vi "Map Tags to Channels.vi"(7 "instance id":string, 8 "error in (no error)":errorcluster, 9 "String Array":string[][](array[string]), 10 "Lines":T1[](array[typedef]), 11 "engine configuration in":refnum<class "engine configuration.lvclass">) -> (0 "error out":errorcluster, 3 "engine configuration out":refnum<class "engine configuration.lvclass">)   [LabVIEW 2018, in "Benchmark PID editor node.lvclass"]
uses:
  Benchmark PID editor node.lvclass
  module/configuration/Line.ctl
  <vilib>/NI/Tag Bus Module Framework/channel/TBM channel.lvclass
  C:/Program Files (x86)/National Instruments/LabVIEW 2018/vi.lib/NI/Tag Bus/tag/tag descriptor.lvclass
  <vilib>/NI/Module Execution Interface/Engine Configuration/engine configuration.lvclass
  <vilib>/NI/Tag Bus/tag/tag descriptor.lvclass/tag descriptor.ctl
  <vilib>/NI/Tag Bus/tag/tag descriptor.lvclass
  module/configuration/Benchmark PID configuration.lvclass
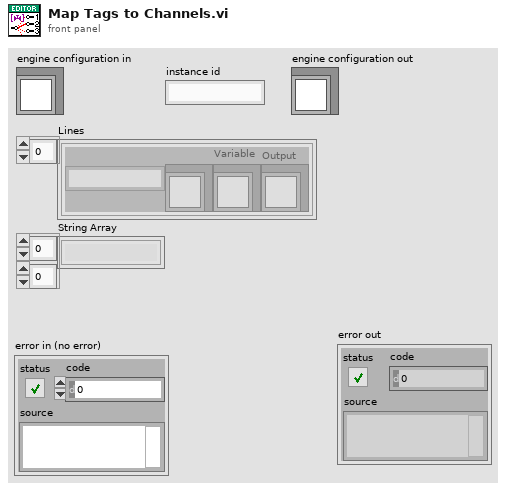
[diagram p1: front panel]
types:
  T1 = typedef "Benchmark PID configuration.lvclass/Line.ctl" = cluster{"PID Name":string, "Setpoint":refnum<class "TBM channel.lvclass">, "Variable":refnum<class "TBM channel.lvclass">, "Output":refnum<class "TBM channel.lvclass">}
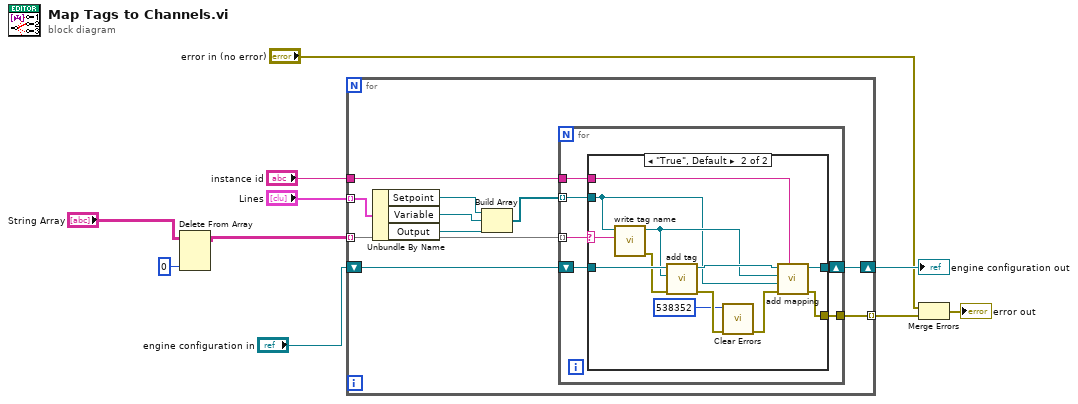
[diagram p0: block diagram]
diagram:
  n1 = Delete From Array(array="String Array", index (col)=0 ("disabled index (col)")) -> (array with subset deleted=w1:string[][])  [unwired: 2 in, 1 out]
  n2 = for {
    tunnel: "Lines" -> [w20] mode=indexing
    tunnel: w1 -> [w15] mode=indexing
    shift-right: [w19] -> w7
    shift-left: "engine configuration in" -> [w16]
    tunnel: "instance id" -> [w18]
    tunnel: [w17] -> w9 mode=indexing
    n3 = Unbundle By Name(w20) -> ("Setpoint"=w14:refnum<class "TBM channel.lvclass">, "Variable"=w12:refnum<class "TBM channel.lvclass">, "Output"=w11:refnum<class "TBM channel.lvclass">)
    n4 = Build Array(w14, w12, w11) -> (w13:refnum<class "TBM channel.lvclass">[])
    n5 = for {
      tunnel: w18 -> [w25]
      tunnel: [w24] -> w17
      tunnel: w13 -> [w22] mode=indexing
      tunnel: w15 -> [w21] mode=indexing
      shift-right: [w26] -> w19
      shift-left: w16 -> [w23]
      n6 = case shown="\"True\", Default" w21 {
        selector: w21 -> [_ w28]
        tunnel: [w27 w39] -> w26
        tunnel: w25 -> [_ w38]
        tunnel: [_ w37] -> w24
        tunnel: w23 -> [w27 w36]
        tunnel: w22 -> [_ w33]
        frame "" {
        }
        frame "True", Default {
          n7 = call <vilib>:"write tag name.vi"("name"=w28, "system tag in"=w33) -> ("error out"=w32:errorcluster, "system tag out"=w34:refnum<class "TBM channel.lvclass">)  [unwired: 8 in]
          n8 = call-dynamic "add tag.vi"("error in"=w32, "tag descriptor"=w34, "engine configuration in"=w36) -> ("error out"=w31:errorcluster, "engine configuration out"=w35:refnum<class "engine configuration.lvclass">)  [unwired: 7 in]
          n9 = call <vilib>:"Clear Errors.vi"("error in (no error)"=w31, "specific error code to clear (0: all)"=538352) -> ("error out"=w30:errorcluster)  [unwired: 4 in, 1 out]
          n10 = call-dynamic "add mapping.vi"("owner ID"=w38, "error in"=w30, "channel"=w33, "tag descriptor"=w34, "engine configuration"=w35) -> ("error out"=w37:errorcluster, "engine configuration out"=w39:refnum<class "engine configuration.lvclass">)  [unwired: 5 in]
        }
      }
    }
  }
  "engine configuration out" <- w7
  n11 = Merge Errors("error in (no error)", w9) -> (→"error out":errorcluster)
